vi "GetHelp.vi"(0 "XRef":T21, 1 "Point":T20, 2 "State In":T13 {"BlockNodeState"."Draw Style" items=["FunctionBlock", "ExpressVI", "Variable", "Elemental I/O", "32x32 Icon", "FunctionBlockCompact"]; "BlockNodeState"."Terminal Data"."Terminal Flags" format="%.0b"}) -> (14 "Standard Help Info":T11, 15 "Detailed Help Info":T8, 16 "Subitem Help Info":T2, 17 "Use Detailed Help?":T1, 18 "Use Subitem Help?":T1)   [LabVIEW 2020, in "Set DDT Attributes.lvlib" / "Set DDT Properties.xnode"]
doc: "Sets the attributes of the dynamic data you wire to <B>Signals In</B>."
uses:
  <vilib>/express/express signal manip/GetorSetDDTAttributes/Set DDT Attributes/Set DDT Properties.xnode
  <vilib>/XNodeSupport/XNodeXNodeRef.ctl
  <vilib>/XNodeSupport/XNodePoint.ctl
  <vilib>/XNodeSupport/XNodeInt.ctl
  <vilib>/express/express signal manip/GetorSetDDTAttributes/Set DDT Attributes/State.ctl
  <vilib>/BlockNodeSupport/BlockNodeState.ctl
  <vilib>/BlockNodeSupport/TerminalData.ctl
  <vilib>/picture/picture.llb/imagedata.ctl
  <vilib>/express/express signal manip/GetorSetDDTAttributes/Shared VIs/Attributes data.ctl
  <vilib>/express/express signal manip/GetorSetDDTAttributes/Shared VIs/Input.ctl
  <vilib>/express/express signal manip/GetorSetDDTAttributes/Shared VIs/Attributes name.ctl
  <vilib>/XNodeSupport/XNodeStandardHelpInfo.ctl
  <vilib>/XNodeSupport/XNodeString.ctl
  <vilib>/XNodeSupport/XNodePath.ctl
  <vilib>/XNodeSupport/XNodeDetailedHelpInfo.ctl
  <vilib>/XNodeSupport/XNodeImage.ctl
  <vilib>/XNodeSupport/XNodeRect32.ctl
  <vilib>/XNodeSupport/XNodeTerms.ctl
  <vilib>/XNodeSupport/XNodeTerm.ctl
  <vilib>/XNodeSupport/XNodeVariant.ctl
  <vilib>/XNodeSupport/XNodeBool.ctl
  <vilib>/XNodeSupport/XNodeSubitemHelpInfo.ctl
  <vilib>/XNodeSupport/NI_XNodeSupport.lvlib
  <vilib>/express/express signal manip/GetorSetDDTAttributes/Shared VIs/GetSetShared.lvlib
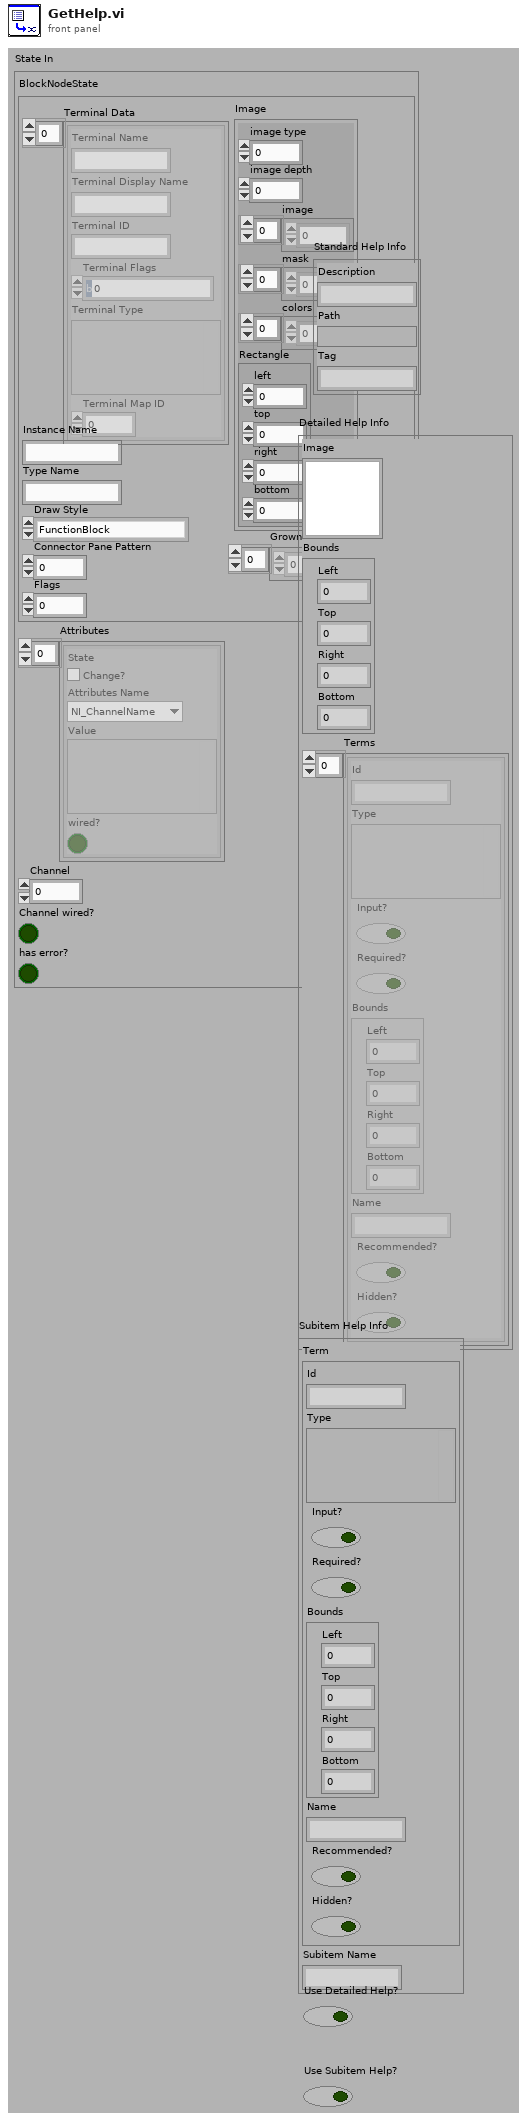
[diagram p1: front panel]
types:
  T1 = typedef "NI_XNodeSupport.lvlib/XNodeBool.ctl" = bool
  T2 = typedef "NI_XNodeSupport.lvlib/XNodeSubitemHelpInfo.ctl" = cluster{"Term":T3, "Subitem Name":T4}
  T3 = typedef "NI_XNodeSupport.lvlib/XNodeTerm.ctl" = cluster{"Id":T4, "Type":T5, "Input?":T1, "Required?":T1, "Bounds":T6, "Name":T4, "Recommended?":T1, "Hidden?":T1}
  T4 = typedef "NI_XNodeSupport.lvlib/XNodeString.ctl" = string
  T5 = typedef "NI_XNodeSupport.lvlib/XNodeVariant.ctl" = variant
  T6 = typedef "NI_XNodeSupport.lvlib/XNodeRect32.ctl" = cluster{"Left":T7, "Top":T7, "Right":T7, "Bottom":T7}
  T7 = typedef "NI_XNodeSupport.lvlib/XNodeInt.ctl" = i32
  T8 = typedef "NI_XNodeSupport.lvlib/XNodeDetailedHelpInfo.ctl" = cluster{"Image":T9, "Bounds":T6, "Terms":T10}
  T9 = typedef "NI_XNodeSupport.lvlib/XNodeImage.ctl" = picture
  T10 = typedef "NI_XNodeSupport.lvlib/XNodeTerms.ctl" = T3[]
  T11 = typedef "NI_XNodeSupport.lvlib/XNodeStandardHelpInfo.ctl" = cluster{"Description":T4, "Path":T12, "Tag":T4}
  T12 = typedef "NI_XNodeSupport.lvlib/XNodePath.ctl" = path
  T13 = typedef "Set DDT Attributes.lvlib/Set DDT Properties.xnode/State.ctl" = cluster{"BlockNodeState":T14, "Attributes":T17[], "Channel":u32, "Channel wired?":bool, "has error?":bool}
  T14 = typedef "BlockNodeState.ctl" = cluster{"Terminal Data":T15[], "Instance Name":string, "Type Name":string, "Draw Style":i32, "Connector Pane Pattern":i32, "Flags":i32, "Grown Terminal List Order":i32[], "Image":T16}
  T15 = typedef "TerminalData.ctl" = cluster{"Terminal Name":string, "Terminal Display Name":string, "Terminal ID":string, "Terminal Flags":i32, "Terminal Type":variant, "Terminal Map ID":i32}
  T16 = typedef "imagedata.ctl" = cluster{"image type":i32, "image depth":i32, "image":u8[], "mask":u8[], "colors":u32[], "Rectangle":cluster{"left":i16, "top":i16, "right":i16, "bottom":i16}}
  T17 = typedef "GetSetShared.lvlib/Attributes data.ctl" = cluster{"State":T18, "Attributes Name":T19, "Value":variant, "wired?":bool}
  T18 = typedef "GetSetShared.lvlib/Input.ctl" = bool
  T19 = typedef "GetSetShared.lvlib/Attributes name.ctl" = enum16{"NI_ChannelName", "NI_ExpIsRelativeTime", "NI_ExpTimeStamp", "NI_ExpStartTimeStamp", "NI_ExpXDimension", "NI_UnitDescription"}
  T20 = typedef "NI_XNodeSupport.lvlib/XNodePoint.ctl" = cluster{"H":T7, "V":T7}
  T21 = typedef "NI_XNodeSupport.lvlib/XNodeXNodeRef.ctl" = refnum<vi>
  T22 = cluster{"Description":string, "Path":path, "Tag":string}
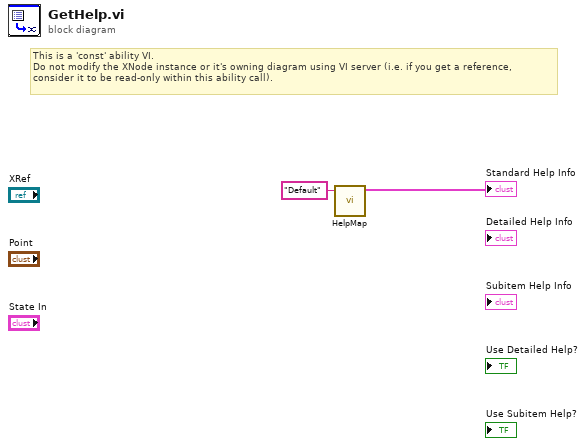
[diagram p0: block diagram]
diagram:
  # "This is a 'const' ability VI.\nDo not modify the XNode instance or it's owning diagram using VI server (i.e. if you get a reference,\nconsider it to be read-only within this ability call)."
  n1 = call <vilib>:"HelpMap.vi"("Standard Help ID"="Default") -> ("Standard Help Info"=→"Standard Help Info":T22)  [unwired: 2 in, 2 out]
